vi "Clear-object.vi"(8 "error in (no error)":errorcluster, 11 "Object ref in":T1) -> (0 "error out":errorcluster)   [LabVIEW 2013, in "MaterialCharacterization.lvlib" / "MC-Main.lvclass"]
uses:
  MC-Main.lvclass
  Object-reference.ctl
  Application-status.ctl
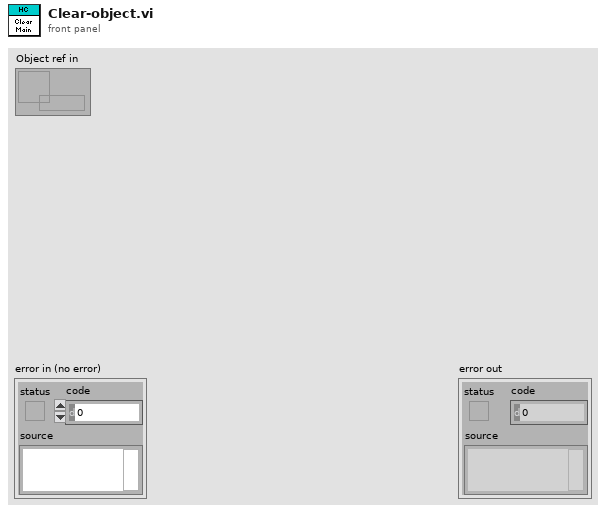
[diagram p1: front panel]
types:
  T1 = typedef "MaterialCharacterization.lvlib/MC-Main.lvclass/Object-reference.ctl" = refnum<data-value>
  T2 = typedef "MaterialCharacterization.lvlib/MC-Main.lvclass/Application-status.ctl" = enum16{"Idle", "Initialized", "Configured", "Activated", "Started", "Paused", "Stopped", "Reset", "Error", "Exited"}
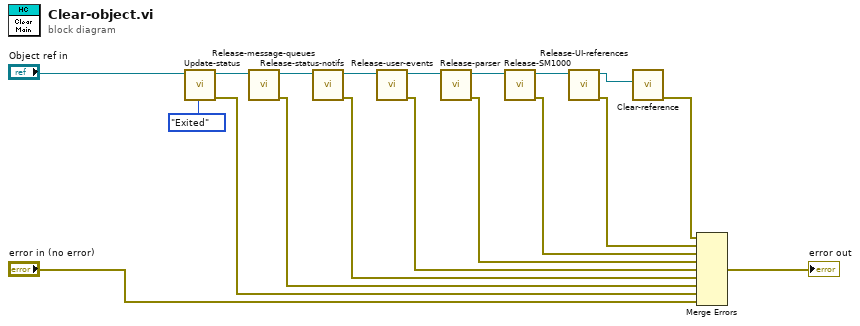
[diagram p0: block diagram]
diagram:
  n1 = call "Update-status.vi"("Status"=Application-status."Exited", "Object ref in"="Object ref in") -> ("error out"=w8:errorcluster, "Object ref out"=w7:T1)  [unwired: 8 in]
  n2 = call "Release-message-queues.vi"("Object ref in"=w7) -> ("error out"=w14:errorcluster, "Object ref out"=w18:T1)  [unwired: 9 in]
  n3 = call "Release-status-notifs.vi"("Object ref in"=w18) -> ("error out"=w13:errorcluster, "Object ref out"=w17:T1)  [unwired: 9 in]
  n4 = call "Release-user-events.vi"("Object ref in"=w17) -> ("error out"=w12:errorcluster, "Object ref out"=w5:T1)  [unwired: 9 in]
  n5 = call "Release-parser.vi"("Object ref in"=w5) -> ("error out"=w1:errorcluster, "Object ref out"=w4:T1)  [unwired: 9 in]
  n6 = call "Release-SM1000.vi"("Object ref in"=w4) -> ("error out"=w2:errorcluster, "Object ref out"=w3:T1)  [unwired: 9 in]
  n7 = call "Release-UI-references.vi"("Object ref in"=w3) -> ("error out"=w11:errorcluster, "Object ref out"=w6:T1)  [unwired: 9 in]
  n8 = call "Clear-reference.vi"("Data ref"=w6) -> ("error out"=w16:errorcluster)  [unwired: 10 in]
  n9 = Merge Errors(w16, w11, w2, w1, w12, w13, w14, w8, "error in (no error)") -> (→"error out":errorcluster)
